vi "Example_USBHub3c.vi"() -> ()   [LabVIEW 2021, in "BrainStem2_LabVIEW_Library.lvlib"]
uses:
  BrainStem2_LabVIEW_Library.lvlib
panel:
  in  "Set Upstream":dbl
  out "PowerC (Port7) - VBus  Current":i32
  out "PowerC (Port 7) - VBus Voltage":i32
  out "Control (Port 6) - VConn Current":i32
  out "Control (Port 6) - VConn Voltage":i32
  out "Control (Port 6) - VBus Current":i32
  out "Control (Port 6) - VBus Voltage":i32
  in  "Port 5 Enable":bool=TRUE
  out "Port 5 - VConn Current":i32
  out "Port 5 - VConn Voltage":i32
  out "Port 5 - VBus Current":i32
  out "Port 5 - VBus Voltage":i32
  in  "Port 4 Enable":bool=TRUE
  out "Port 4 - VConn Current":i32
  out "Port 4 - VConn Voltage":i32
  out "Port 4 - VBus Current":i32
  out "Port 4 - VBus Voltage":i32
  in  "Port 3 Enable":bool=TRUE
  out "Port 3 - VConn Current":i32
  out "Port 3 - VConn Voltage":i32
  out "Port 3 - VBus Current":i32
  out "Port 3 - VBus Voltage":i32
  in  "Port 2 Enable":bool=TRUE
  out "Port 2 - VConn Current":i32
  out "Port 2 - VConn Voltage":i32
  out "Port 2 - VBus Current":i32
  out "Port 2 - VBus Voltage":i32
  in  "Port 1 Enable":bool=TRUE
  out "Port 1 - VConn Current":i32
  out "Port 1 - VConn Voltage":i32
  out "Port 1 - VBus Current":i32
  out "Port 1 - VBus Voltage":i32
  out "Upstream Port":dbl
  in  "Port 0 Enable":bool=TRUE
  out "Port 0 - VConn Current":i32
  out "Port 0 - VConn Voltage":i32
  out "Port 0 - VBus Current":i32
  out "Port 0 - VBus Voltage":i32
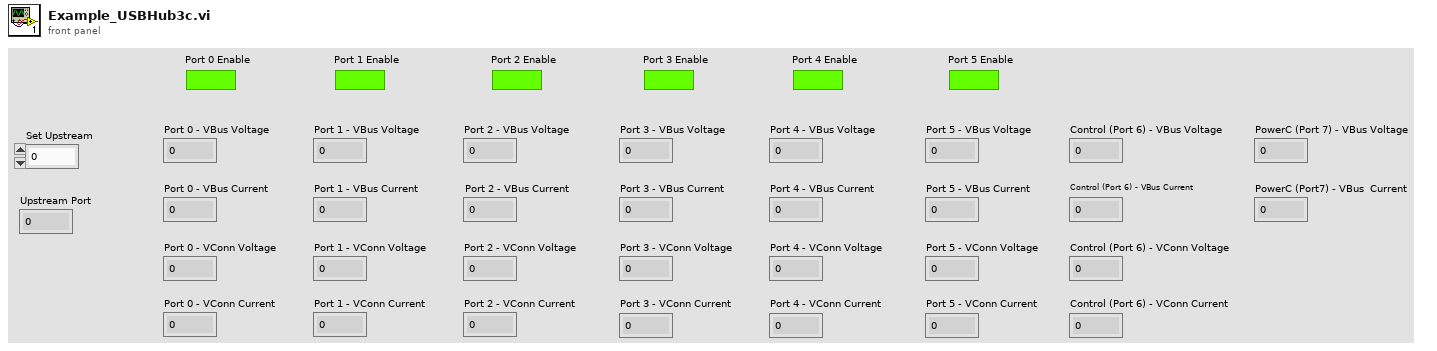
[diagram p1: front panel]
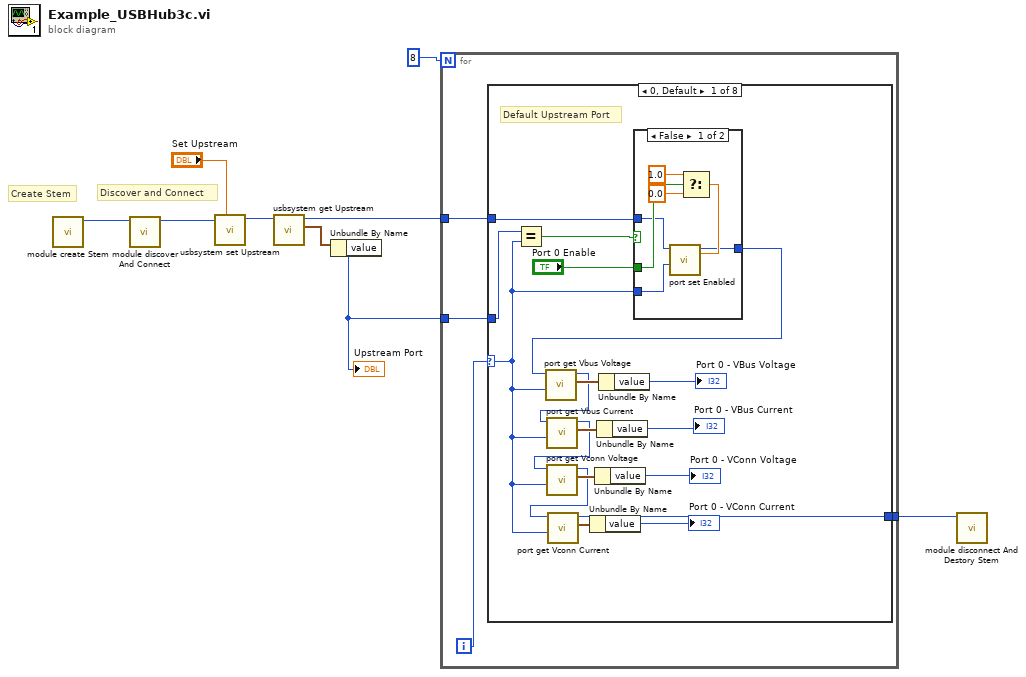
[diagram p0: block diagram]
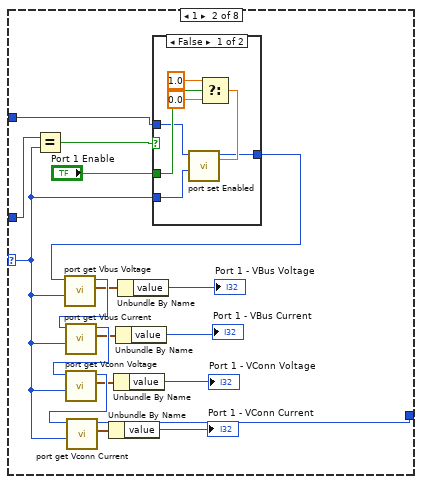
[diagram p3: hidden frame]
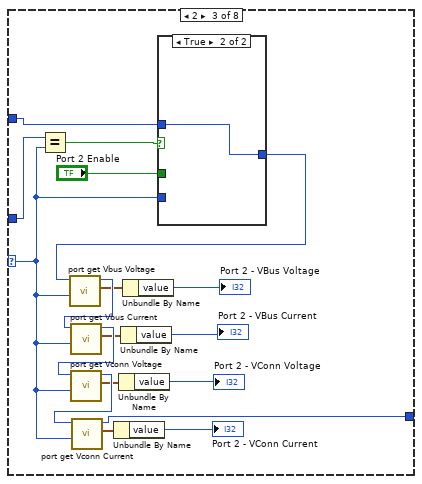
[diagram p5: hidden frame]
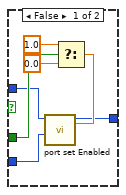
[diagram p6: hidden frame]
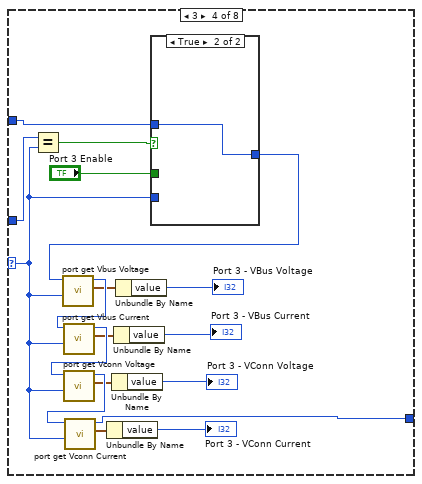
[diagram p7: hidden frame]
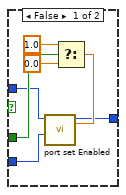
[diagram p8: hidden frame]
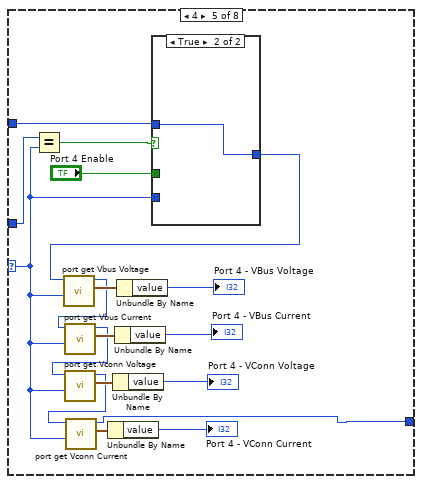
[diagram p9: hidden frame]
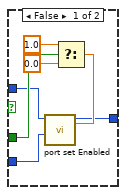
[diagram p10: hidden frame]
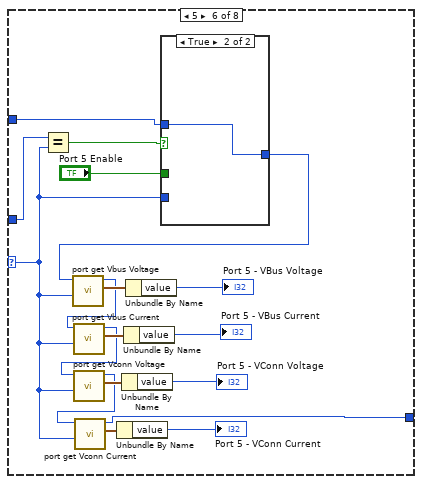
[diagram p11: hidden frame]
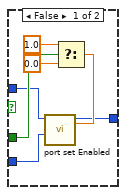
[diagram p12: hidden frame]
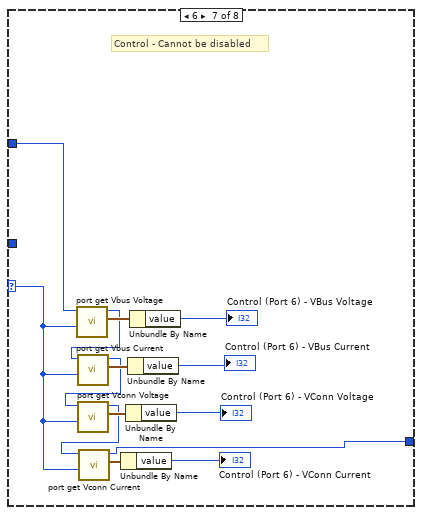
[diagram p13: hidden frame]
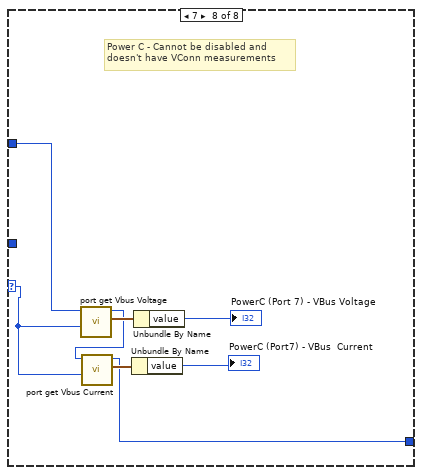
[diagram p14: hidden frame]
diagram:
  # "Discover and Connect"
  # "Create Stem"
  n1 = call "module create Stem.vi"() -> ("id out"=w9:u32)  [unwired: 9 in, 2 out]
  n2 = call "module discover And Connect.vi"("id"=w9) -> ("id out"=w2:u32)  [unwired: 8 in, 2 out]
  n3 = call "usbsystem set Upstream.vi"("port"="Set Upstream", "id"=w2) -> ("id out"=w1:u32)  [unwired: 7 in, 2 out]
  n4 = call "usbsystem get Upstream.vi"("id"=w1) -> ("result out"=w8:cluster{"value":i32, "error":i32}, "id out"=w6:u32)  [unwired: 8 in, 1 out]
  n5 = Unbundle By Name(w8) -> ("value"=w5:i32)
  "Upstream Port" <- w5
  n6 = for {
    N: 8 -> [_]
    tunnel: w5 -> [w12]
    tunnel: w6 -> [w11]
    tunnel: [w10] -> w4
    i -> [w13]
    n7 = case shown="0, Default" w13 {
      selector: w13 -> [w15 w42 w67 w93 w119 w145 w171 w184]
      tunnel: w12 -> [w23 w43 w68 w94 w120 w146 _ _]
      tunnel: w11 -> [w20 w41 w69 w95 w121 w147 w172 w185]
      tunnel: [w14 w40 w66 w92 w118 w144 w170 w186] -> w10
      frame 0, Default {
        # "Default Upstream Port"
        n8 = Equal?(x=w23, y=w15) -> (x = y?=w22:bool)
        n9 = case shown="False" w22 {
          tunnel: w15 -> [w38 _]
          tunnel: "Port 0 Enable" -> [w37 _]
          tunnel: w20 -> [w33 w39]
          tunnel: [w32 w39] -> w19
          frame False {
            n10 = Select(t=1.0, s=w37, f=0.0) -> (s? t:f=w34:dbl)
            n11 = call "port set Enabled.vi"("enable"=w34, "index"=w38, "id"=w33) -> ("id out"=w32:u32)  [unwired: 6 in, 2 out]
          }
          frame True {
          }
        }
        n12 = call "port get Vbus Voltage.vi"("index"=w15, "id"=w19) -> ("result out"=w31:cluster{"value":i32, "error":i32}, "id out"=w18:u32)  [unwired: 7 in, 1 out]
        n13 = call "port get Vbus Current.vi"("index"=w15, "id"=w18) -> ("result out"=w29:cluster{"value":i32, "error":i32}, "id out"=w17:u32)  [unwired: 7 in, 1 out]
        n14 = call "port get Vconn Voltage.vi"("index"=w15, "id"=w17) -> ("result out"=w28:cluster{"value":i32, "error":i32}, "id out"=w16:u32)  [unwired: 7 in, 1 out]
        n15 = call "port get Vconn Current.vi"("index"=w15, "id"=w16) -> ("result out"=w27:cluster{"value":i32, "error":i32}, "id out"=w14:u32)  [unwired: 7 in, 1 out]
        n16 = Unbundle By Name(w27) -> ("value"=→"Port 0 - VConn Current":i32)
        n17 = Unbundle By Name(w28) -> ("value"=→"Port 0 - VConn Voltage":i32)
        n18 = Unbundle By Name(w29) -> ("value"=→"Port 0 - VBus Current":i32)
        n19 = Unbundle By Name(w31) -> ("value"=→"Port 0 - VBus Voltage":i32)
      }
      frame 1 {
        n20 = Equal?(x=w43, y=w42) -> (x = y?=w52:bool)
        n21 = case shown="False" w52 {
          tunnel: w42 -> [w64 _]
          tunnel: "Port 1 Enable" -> [w63 _]
          tunnel: w41 -> [w59 w65]
          tunnel: [w58 w65] -> w54
          frame False {
            n22 = Select(t=1.0, s=w63, f=0.0) -> (s? t:f=w60:dbl)
            n23 = call "port set Enabled.vi"("enable"=w60, "index"=w64, "id"=w59) -> ("id out"=w58:u32)  [unwired: 6 in, 2 out]
          }
          frame True {
          }
        }
        n24 = call "port get Vbus Voltage.vi"("index"=w42, "id"=w54) -> ("result out"=w44:cluster{"value":i32, "error":i32}, "id out"=w55:u32)  [unwired: 7 in, 1 out]
        n25 = call "port get Vbus Current.vi"("index"=w42, "id"=w55) -> ("result out"=w46:cluster{"value":i32, "error":i32}, "id out"=w56:u32)  [unwired: 7 in, 1 out]
        n26 = call "port get Vconn Voltage.vi"("index"=w42, "id"=w56) -> ("result out"=w47:cluster{"value":i32, "error":i32}, "id out"=w57:u32)  [unwired: 7 in, 1 out]
        n27 = call "port get Vconn Current.vi"("index"=w42, "id"=w57) -> ("result out"=w48:cluster{"value":i32, "error":i32}, "id out"=w40:u32)  [unwired: 7 in, 1 out]
        n28 = Unbundle By Name(w48) -> ("value"=→"Port 1 - VConn Current":i32)
        n29 = Unbundle By Name(w47) -> ("value"=→"Port 1 - VConn Voltage":i32)
        n30 = Unbundle By Name(w46) -> ("value"=→"Port 1 - VBus Current":i32)
        n31 = Unbundle By Name(w44) -> ("value"=→"Port 1 - VBus Voltage":i32)
      }
      frame 2 {
        n32 = Equal?(x=w68, y=w67) -> (x = y?=w78:bool)
        n33 = case shown="True" w78 {
          tunnel: w67 -> [w90 _]
          tunnel: "Port 2 Enable" -> [w89 _]
          tunnel: w69 -> [w85 w91]
          tunnel: [w84 w91] -> w80
          frame False {
            n34 = Select(t=1.0, s=w89, f=0.0) -> (s? t:f=w86:dbl)
            n35 = call "port set Enabled.vi"("enable"=w86, "index"=w90, "id"=w85) -> ("id out"=w84:u32)  [unwired: 6 in, 2 out]
          }
          frame True {
          }
        }
        n36 = call "port get Vbus Voltage.vi"("index"=w67, "id"=w80) -> ("result out"=w70:cluster{"value":i32, "error":i32}, "id out"=w81:u32)  [unwired: 7 in, 1 out]
        n37 = call "port get Vbus Current.vi"("index"=w67, "id"=w81) -> ("result out"=w72:cluster{"value":i32, "error":i32}, "id out"=w82:u32)  [unwired: 7 in, 1 out]
        n38 = call "port get Vconn Voltage.vi"("index"=w67, "id"=w82) -> ("result out"=w73:cluster{"value":i32, "error":i32}, "id out"=w83:u32)  [unwired: 7 in, 1 out]
        n39 = call "port get Vconn Current.vi"("index"=w67, "id"=w83) -> ("result out"=w74:cluster{"value":i32, "error":i32}, "id out"=w66:u32)  [unwired: 7 in, 1 out]
        n40 = Unbundle By Name(w74) -> ("value"=→"Port 2 - VConn Current":i32)
        n41 = Unbundle By Name(w73) -> ("value"=→"Port 2 - VConn Voltage":i32)
        n42 = Unbundle By Name(w72) -> ("value"=→"Port 2 - VBus Current":i32)
        n43 = Unbundle By Name(w70) -> ("value"=→"Port 2 - VBus Voltage":i32)
      }
      frame 3 {
        n44 = Equal?(x=w94, y=w93) -> (x = y?=w104:bool)
        n45 = case shown="True" w104 {
          tunnel: w93 -> [w116 _]
          tunnel: "Port 3 Enable" -> [w115 _]
          tunnel: w95 -> [w111 w117]
          tunnel: [w110 w117] -> w106
          frame False {
            n46 = Select(t=1.0, s=w115, f=0.0) -> (s? t:f=w112:dbl)
            n47 = call "port set Enabled.vi"("enable"=w112, "index"=w116, "id"=w111) -> ("id out"=w110:u32)  [unwired: 6 in, 2 out]
          }
          frame True {
          }
        }
        n48 = call "port get Vbus Voltage.vi"("index"=w93, "id"=w106) -> ("result out"=w96:cluster{"value":i32, "error":i32}, "id out"=w107:u32)  [unwired: 7 in, 1 out]
        n49 = call "port get Vbus Current.vi"("index"=w93, "id"=w107) -> ("result out"=w98:cluster{"value":i32, "error":i32}, "id out"=w108:u32)  [unwired: 7 in, 1 out]
        n50 = call "port get Vconn Voltage.vi"("index"=w93, "id"=w108) -> ("result out"=w99:cluster{"value":i32, "error":i32}, "id out"=w109:u32)  [unwired: 7 in, 1 out]
        n51 = call "port get Vconn Current.vi"("index"=w93, "id"=w109) -> ("result out"=w100:cluster{"value":i32, "error":i32}, "id out"=w92:u32)  [unwired: 7 in, 1 out]
        n52 = Unbundle By Name(w100) -> ("value"=→"Port 3 - VConn Current":i32)
        n53 = Unbundle By Name(w99) -> ("value"=→"Port 3 - VConn Voltage":i32)
        n54 = Unbundle By Name(w98) -> ("value"=→"Port 3 - VBus Current":i32)
        n55 = Unbundle By Name(w96) -> ("value"=→"Port 3 - VBus Voltage":i32)
      }
      frame 4 {
        n56 = Equal?(x=w120, y=w119) -> (x = y?=w127:bool)
        n57 = case shown="True" w127 {
          tunnel: w119 -> [w142 _]
          tunnel: "Port 4 Enable" -> [w141 _]
          tunnel: w121 -> [w137 w143]
          tunnel: [w136 w143] -> w125
          frame False {
            n58 = Select(t=1.0, s=w141, f=0.0) -> (s? t:f=w138:dbl)
            n59 = call "port set Enabled.vi"("enable"=w138, "index"=w142, "id"=w137) -> ("id out"=w136:u32)  [unwired: 6 in, 2 out]
          }
          frame True {
          }
        }
        n60 = call "port get Vbus Voltage.vi"("index"=w119, "id"=w125) -> ("result out"=w135:cluster{"value":i32, "error":i32}, "id out"=w124:u32)  [unwired: 7 in, 1 out]
        n61 = call "port get Vbus Current.vi"("index"=w119, "id"=w124) -> ("result out"=w133:cluster{"value":i32, "error":i32}, "id out"=w123:u32)  [unwired: 7 in, 1 out]
        n62 = call "port get Vconn Voltage.vi"("index"=w119, "id"=w123) -> ("result out"=w132:cluster{"value":i32, "error":i32}, "id out"=w122:u32)  [unwired: 7 in, 1 out]
        n63 = call "port get Vconn Current.vi"("index"=w119, "id"=w122) -> ("result out"=w131:cluster{"value":i32, "error":i32}, "id out"=w118:u32)  [unwired: 7 in, 1 out]
        n64 = Unbundle By Name(w131) -> ("value"=→"Port 4 - VConn Current":i32)
        n65 = Unbundle By Name(w132) -> ("value"=→"Port 4 - VConn Voltage":i32)
        n66 = Unbundle By Name(w133) -> ("value"=→"Port 4 - VBus Current":i32)
        n67 = Unbundle By Name(w135) -> ("value"=→"Port 4 - VBus Voltage":i32)
      }
      frame 5 {
        n68 = Equal?(x=w146, y=w145) -> (x = y?=w153:bool)
        n69 = case shown="True" w153 {
          tunnel: w145 -> [w168 _]
          tunnel: "Port 5 Enable" -> [w167 _]
          tunnel: w147 -> [w163 w169]
          tunnel: [w162 w169] -> w151
          frame False {
            n70 = Select(t=1.0, s=w167, f=0.0) -> (s? t:f=w164:dbl)
            n71 = call "port set Enabled.vi"("enable"=w164, "index"=w168, "id"=w163) -> ("id out"=w162:u32)  [unwired: 6 in, 2 out]
          }
          frame True {
          }
        }
        n72 = call "port get Vbus Voltage.vi"("index"=w145, "id"=w151) -> ("result out"=w161:cluster{"value":i32, "error":i32}, "id out"=w150:u32)  [unwired: 7 in, 1 out]
        n73 = call "port get Vbus Current.vi"("index"=w145, "id"=w150) -> ("result out"=w159:cluster{"value":i32, "error":i32}, "id out"=w149:u32)  [unwired: 7 in, 1 out]
        n74 = call "port get Vconn Voltage.vi"("index"=w145, "id"=w149) -> ("result out"=w158:cluster{"value":i32, "error":i32}, "id out"=w148:u32)  [unwired: 7 in, 1 out]
        n75 = call "port get Vconn Current.vi"("index"=w145, "id"=w148) -> ("result out"=w157:cluster{"value":i32, "error":i32}, "id out"=w144:u32)  [unwired: 7 in, 1 out]
        n76 = Unbundle By Name(w157) -> ("value"=→"Port 5 - VConn Current":i32)
        n77 = Unbundle By Name(w158) -> ("value"=→"Port 5 - VConn Voltage":i32)
        n78 = Unbundle By Name(w159) -> ("value"=→"Port 5 - VBus Current":i32)
        n79 = Unbundle By Name(w161) -> ("value"=→"Port 5 - VBus Voltage":i32)
      }
      frame 6 {
        # "Control - Cannot be disabled"
        n80 = call "port get Vbus Voltage.vi"("index"=w171, "id"=w172) -> ("result out"=w183:cluster{"value":i32, "error":i32}, "id out"=w175:u32)  [unwired: 7 in, 1 out]
        n81 = call "port get Vbus Current.vi"("index"=w171, "id"=w175) -> ("result out"=w181:cluster{"value":i32, "error":i32}, "id out"=w174:u32)  [unwired: 7 in, 1 out]
        n82 = call "port get Vconn Voltage.vi"("index"=w171, "id"=w174) -> ("result out"=w180:cluster{"value":i32, "error":i32}, "id out"=w173:u32)  [unwired: 7 in, 1 out]
        n83 = call "port get Vconn Current.vi"("index"=w171, "id"=w173) -> ("result out"=w179:cluster{"value":i32, "error":i32}, "id out"=w170:u32)  [unwired: 7 in, 1 out]
        n84 = Unbundle By Name(w179) -> ("value"=→"Control (Port 6) - VConn Current":i32)
        n85 = Unbundle By Name(w180) -> ("value"=→"Control (Port 6) - VConn Voltage":i32)
        n86 = Unbundle By Name(w181) -> ("value"=→"Control (Port 6) - VBus Current":i32)
        n87 = Unbundle By Name(w183) -> ("value"=→"Control (Port 6) - VBus Voltage":i32)
      }
      frame 7 {
        # "Power C - Cannot be disabled and \ndoesn't have VConn measurements"
        n88 = call "port get Vbus Voltage.vi"("index"=w184, "id"=w185) -> ("result out"=w191:cluster{"value":i32, "error":i32}, "id out"=w187:u32)  [unwired: 7 in, 1 out]
        n89 = call "port get Vbus Current.vi"("index"=w184, "id"=w187) -> ("result out"=w189:cluster{"value":i32, "error":i32}, "id out"=w186:u32)  [unwired: 7 in, 1 out]
        n90 = Unbundle By Name(w189) -> ("value"=→"PowerC (Port7) - VBus  Current":i32)
        n91 = Unbundle By Name(w191) -> ("value"=→"PowerC (Port 7) - VBus Voltage":i32)
      }
    }
  }
  n92 = call "module disconnect And Destory Stem.vi"("id"=w4) -> ()  [unwired: 8 in, 3 out]
